vi "AlliGator Load SS1 FLI Dataset Information.vi"(8 "error in (no error)":errorcluster, 10 "Laser Period":dbl[unit], 11 "Image Folder":path) -> (0 "error out":errorcluster, 1 "Data Description":string, 2 "Metadata":string, 3 "FLI Data File Information":T1)   [LabVIEW 2021, in "AlliGator Files.lvlib"]
doc: "Loads data information from SS1 dataset."
uses:
  AlliGator Files.lvlib
  AlliGator FLI Data File Information.ctl
  Phasor/Phasor Fluorescence Lifetime Parameters v3.ctl
  AlliGator FLI Dataset Type.ctl
  AlliGator Settings List.ctl
  SwissSPAD/SwissSPAD 1 Extended Dataset Information.ctl
  SwissSPAD/SwissSPAD1 File Information.ctl
  AlliGator Load Single Gate Image from SS1 Dataset.vi
  AlliGator HDF5.lvlib
  Time/Time.lvlib
  SwissSPAD/SwissSPAD.lvlib
  AlliGator Settings.lvlib
  Phasor/Phasor.lvlib
panel:
  out "Header Size":i64
  # "see the AlliGator License on the block diagram (Ctrl+E or Window:Show Block Diagram)"
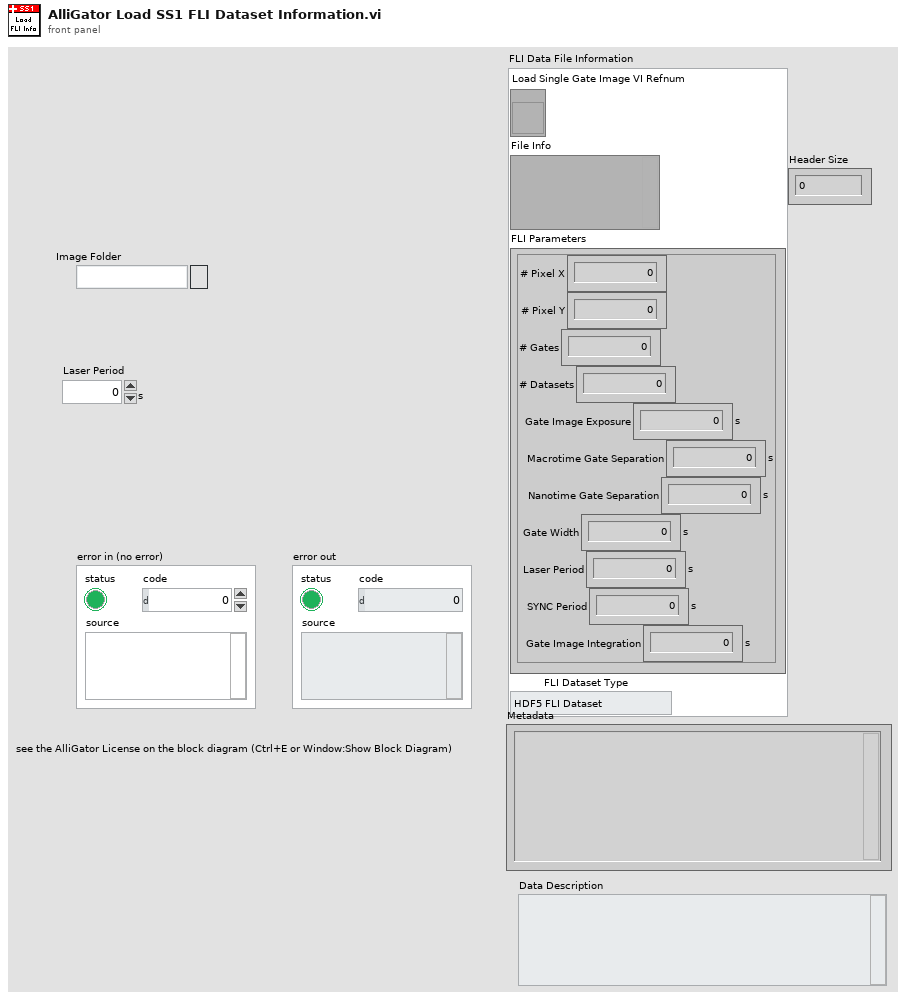
[diagram p1: front panel]
types:
  T1 = typedef "AlliGator HDF5.lvlib/AlliGator FLI Data File Information.ctl" = cluster{"Load Single Gate Image VI Refnum":refnum<vi>, "File Info":variant, "FLI Parameters":T2, "FLI Dataset Type":T3}
  T2 = typedef "Phasor.lvlib/Phasor Fluorescence Lifetime Parameters v3.ctl" = cluster{"# Pixel X":i32, "# Pixel Y":i32, "# Gates":i32, "# Datasets":i32, "Gate Image Exposure":dbl[unit], "Macrotime Gate Separation":dbl[unit], "Nanotime Gate Separation":dbl[unit], "Gate Width":dbl[unit], "Laser Period":dbl[unit], "SYNC Period":dbl[unit], "Gate Image Integration":dbl[unit]}
  T3 = typedef "AlliGator Files.lvlib/AlliGator FLI Dataset Type.ctl" = enum16{"HDF5 FLI Dataset", "Gate Image Folder", ".sdt FLI Dataset (Becker & Hickl)", ".ptu FLI Dataset (PicoQuant)", "SS1 FLI Dataset", "SS2 FLI Dataset", "I/m/phi Dataset", ".bin FLI Dataset (PicoQuant Binned)", ".bin FLI Dataset (Piccolo Binned)"}
  T4 = typedef "SwissSPAD.lvlib/SwissSPAD 1 Extended Dataset Information.ctl" = cluster{"File Path":path, "Data Offset (in bytes)":i64, "# Bytes/Pixel":i32, "# Pixel X":i32, "# Pixel Y":i32, "SwissSPAD1 File Information":T5}
  T5 = typedef "SwissSPAD.lvlib/SwissSPAD1 File Information.ctl" = cluster{"SPAD Off Pattern":u64, "Recharge Pattern":u64, "Gate Pattern":u64, "Pattern Length":u32, "# Repetitions":u32, "Initial Macro Shift":u32, "Initial Micro Shift":u32, "VOP Voltage":dbl, "Top Gate Voltage":dbl, "Bias Voltage":dbl, "# Readouts/Frame":u32, "Scan Start (step unit)":u32, "Scan Increment (step unit)":u32, "# Frames":u32, "Note":string}
  T6 = typedef "AlliGator Settings.lvlib/AlliGator Settings List.ctl" = enum16{"GUI:Visible Settings Tab", "GUI:Last Run Version", "Source Image:Use Image Histogram for Contrast", "Source Image:Low Count Pixels Rejection Options", "Source Image:High Count Pixels Rejection Options", "Source Image:Use Image Brightness", "Source Image:Blend Overlay with Image Background", "Source Image:Use Fixed ROI Diameter", "Source Image:ROI Diameter", "Source Image:ROI Center Color", "Source Image:Peak Threshold", "Source Image:Intensity Threshold", "Source Image:Image Binning Options", "Source Image:Image Smoothing Options", "Source Image:Image Histogram Active", "Source Image:Invert Binary Mask", "Source Image:Hot Pixel Removal", "Source Image:Overlay Analyzed ROI Center", "Source Image:Auto-Adjust Contrast", "Source Image:Histogram Lower Percentile", "Source Image:Histogram Upper Percentile", "Source Image:Save Source Image", "Source Image:Scale Bar Options", "Source Image:Image Resolution (Pixel Size)", "Source Image:Flatfield Correction", "Source Image:Show Dead Left Columns Correction", "Source Image:Dead Left Columns Correction", "Source Image:Image Pre-Processing Operations Order", "Data Information:Gate Width", "Data Information:Nanotime Gate Separation", "Data Information:Macrotime Gate Separation", "Data Information:Gate Step", "Data Information:# Gates", "Data Information:Gate Image Exposure", "Data Information:Gate Image Integration", "Data Information:Gates to Skip", "Data Information:Gates to Keep", "Data Information:Define Gates to", "Data Information:Channel Name", "Data Information:Available Channel Names", "Data Information:Channel Arithmetic", "Data Information:Background File Subtraction", "Data Information:Background File", "Data Information:Background Scaling Factor", "Data Information:Background Pile-up Correction", "Data Information:Background Pixel Well Capacity", "Data Information:Laser Period", "Data Information:SYNC Period", "Data Information:Pile-up Correction", "Data Information:Pixel Well Capacity", "Data Information:Dataset Scaling Factor", "Fluorescence Decay_Decay Pre-Processing:Reverse Gates", "Fluorescence Decay_Decay Pre-Processing:Verbose Decay Pre-Processing", "Fluorescence Decay_Decay Pre-Processing:Use Decay Pre-Processing", "Fluorescence Decay_Decay Pre-Processing:Background Subtraction", "Fluorescence Decay_Decay Pre-Processing:Background Definition Range", "Fluorescence Decay_Decay Pre-Processing:Baseline Subtraction Method", "Fluorescence Decay_Decay Pre-Processing:Decay Pre-Processing Operations Order", "Fluorescence Decay_Decay Pre-Processing:Smoothing Parameter", "Fluorescence Decay_Decay Pre-Processing:Shift Decay", "Fluorescence Decay_Decay Pre-Processing:Decay Shift Parameters", "Fluorescence Decay_Decay Pre-Processing:Fold Decay", "Fluorescence Decay_Decay Pre-Processing:# Folds", "Fluorescence Decay_Decay Pre-Processing:1-Normalize Decay", "Fluorescence Decay_Decay Pre-Processing:[0-1]-Normalize Decay", "Fluorescence Decay_Decay Pre-Processing:Smoothen Decay", "Fluorescence Decay_Decay Pre-Processing:Extrapolate Decay", "Fluorescence Decay_Decay Pre-Processing:Use Periodicity", "Fluorescence Decay_Decay Pre-Processing:Use Cursors", "Fluorescence Decay_Decay Pre-Processing:Tail Fraction", "Fluorescence Decay_Decay Pre-Processing:Head Fraction", "Fluorescence Decay_Decay Pre-Processing:Additional Points", "Fluorescence Decay_Decay Pre-Processing:Straighten Decay", "Fluorescence Decay_Decay Pre-Processing:Constant Background", "Fluorescence Decay_Decay Pre-Processing:Pixel-Normalize Decay", "Fluorescence Decay_Advanced Analysis:Extract IRF instead of Decay", "Fluorescence Decay_Advanced Analysis:IRF Extraction Options", "Fluorescence Decay_Advanced Analysis:IRF Optimization Options", "Fluorescence Decay_Advanced Analysis:Square Pulse Options", "Fluorescence Decay_Advanced Analysis:IRF Order", "Fluorescence Decay_Advanced Analysis:IRF Time Constants", "Fluorescence Decay_Advanced Analysis:Wavelet Analysis Options", "Fluorescence Decay_Advanced Analysis:Average Lifetime Options", "Fluorescence Decay_Fit Options:Fit Options", "Fluorescence Decay_Fit Options:Use Legacy Fitting Approach", "Fluorescence Decay_Fit Options:Use Data Information Laser Period", "Fluorescence Decay_Fit Parameters:Displayed Fit Parameters", "Fluorescence Decay_Fit Parameters:Fit Parameter Constraints", "Fluorescence Decay_Fit Parameters:Export Tabulated Results", "Fluorescence Decay_Fit Parameters:MLE Baseline Offset Type", "Fluorescence Decay_Fit Parameters:MLE Baseline Offset", "Fluorescence Decay_Fit Parameters:Guess Parameter Names", "Fluorescence Decay_Fit Parameters:Guess Parameter Values", "Fluorescence Decay_Fit Parameters:Guess Parameters Options", "Fluorescence Decay_Styles:Show Last Decay Only", "Fluorescence Decay_Styles:Decay Graph Color Array", "Fluorescence Decay:Decay Graph Active", "Fluorescence Decay Statistics:Min Peak Value", "Fluorescence Decay Statistics:Reject Low Decay Peak Pixels", "Fluorescence Decay Statistics:Reject High Decay Peak Pixels", "Fluorescence Decay Statistics:Max Peak Value", "Time Traces:Use File Timestamp", "Time Traces:Time Step", "Time Traces:Use Intensity Correction File", "Time Traces:Intensity Correction File", "Phasor Plot:Phasor Plot Smoothing Options", "Phasor Plot:Phasor Plot Size", "Phasor Plot:Phasor Plot Graphics Options", "Phasor Plot:Cumulative Phasor Plot", "Phasor Plot:Use Phasor Brightness", "Phasor Plot:Blend Overlay with Phasor Background", "Phasor Plot:Save Phasor Plot", "Phasor Plot:Show References", "Phasor Plot:Phasor Ratio Decay Range", "Phasor Plot:Exponential Fading", "Phasor Plot:Phasor Ratio Reference Colors", "Phasor Plot:Reference Radius", "Phasor Plot:Show Color Map Vertices", "Phasor Plot:Phasor Plot Active", "Phasor Plot:Phasor Ratio Color Map Type", "Phasor Plot:Phasor Ratio Color Map", "Phasor Plot:Phasor Ratio Display Range", "Phasor Plot:Selected Image ROI(s)", "Phasor Plot:All Image ROIs", "Phasor Plot:Selected Phasor Plot ROI(s)", "Phasor Plot:All Phasor Plot ROIs", "Phasor Plot:Phasor Ratio Color-Coded Quantity", "Phasor Plot:Store Phasor Harmonics", "Phasor Plot:Draw Reference Segment", "Phasor Plot:User-Defined Quantity", "Phasor Graph:Phasor Frequency", "Phasor Graph:Phasor Ratio Type", "Phasor Graph:Pixel-level Phasor Computation", "Phasor Graph:Save Phasor Graph", "Phasor Graph:Phasor Graph Active", "Phasor Graph:Phasor SDV Options", "Phasor Calibration:Use Backup Calibration if needed", "Phasor Graph:Define Shortest Lifetime as", "Phasor Calibration:Backup Calibration Type", "Phasor Calibration:Calibration Type", "Phasor Calibration:Calibration Lifetime", "Phasor Calibration:Calibration Map Algorithm", "Single-Exponential Phasor Locus (SEPL):Gate Parameters", "Single-Exponential Phasor Locus (SEPL):User-defined Gate", "Single-Exponential Phasor Locus (SEPL):User-defined IRF", "Single-Exponential Phasor Locus (SEPL):Phasor Parameters", "Single-Exponential Phasor Locus (SEPL):Decay & IRF Parameters", "Single-Exponential Phasor Locus (SEPL):Display Parameters", "Lifetime Analysis:Decay Analysis Parameters", "Lifetime Analysis:Lifetime Map Active", "Plugins:Python Settings", "Miscellaneous:Verbose Mode", "Miscellaneous:Beep after Script", "Miscellaneous:Saved Image File Format", "Miscellaneous:Exported Gate Image Settings", "Miscellaneous:Include Loading in Timing", "Miscellaneous:Verbose Settings Mode", "Miscellaneous:Histogram Options", "Miscellaneous:Beep on Error", "Miscellaneous:# Logical Processors Used", "Miscellaneous:ROI Description Max Characters", "Miscellaneous:Verbose Error Mode", "Miscellaneous:Transparent Mask Color"}
  T7 = enum16{"big-endian, network order", "native, host order", "little-endian"}
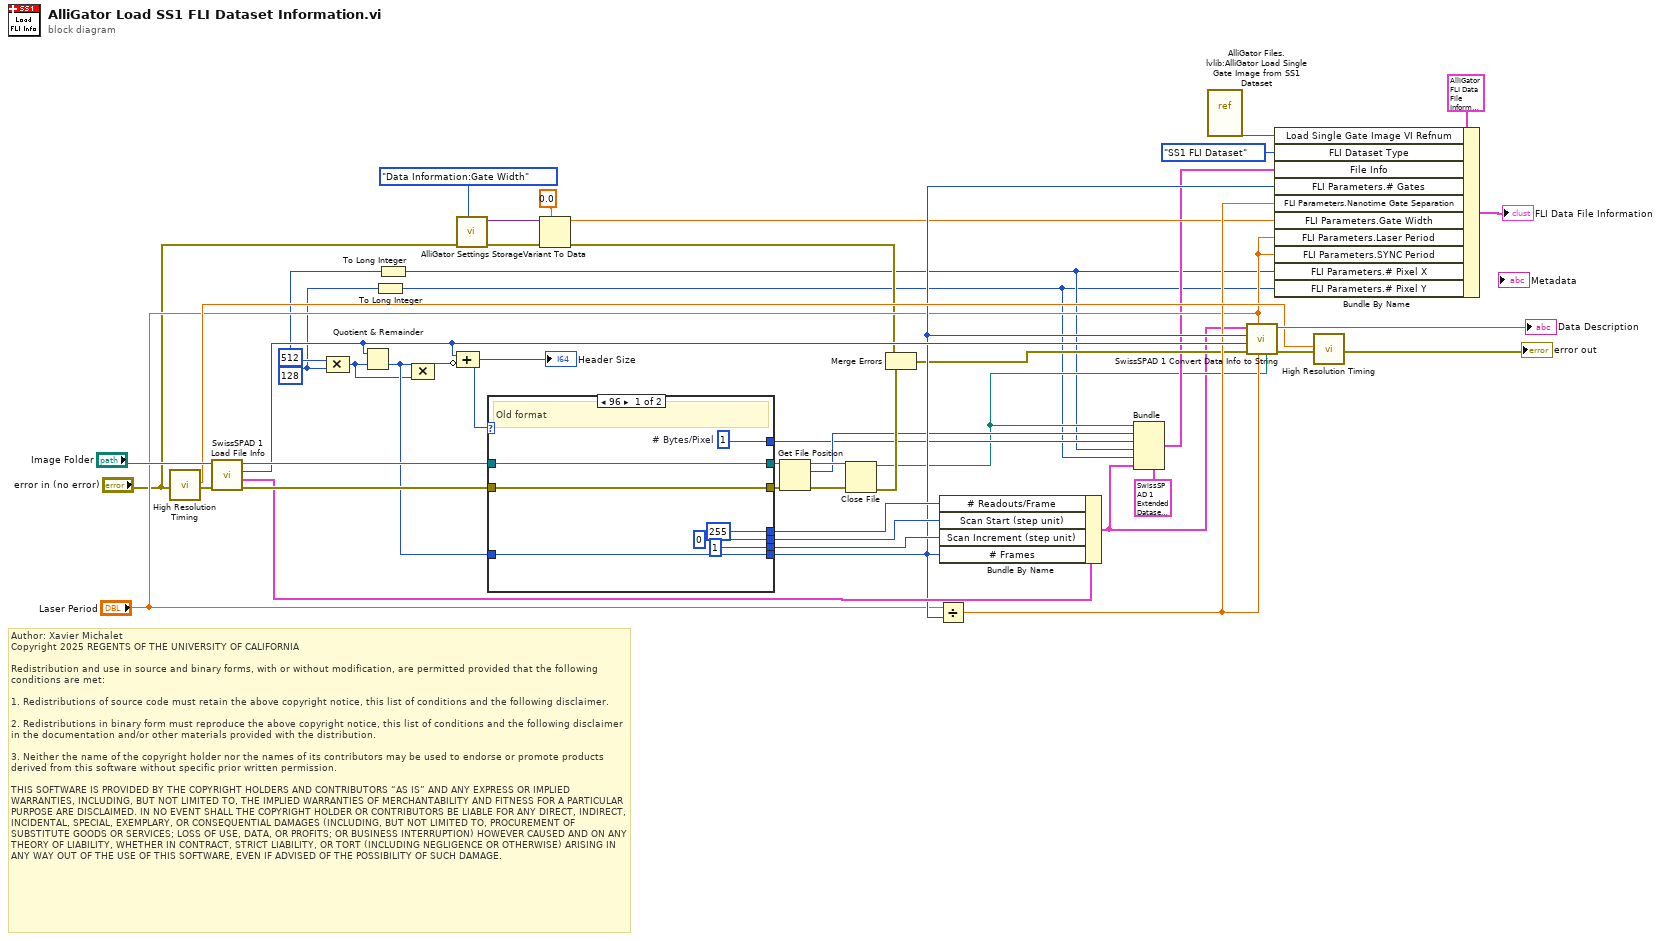
[diagram p0: block diagram]
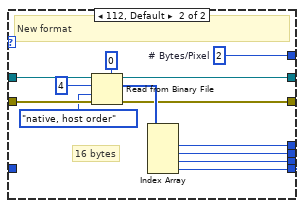
[diagram p2: hidden frame]
diagram:
  w3 = i64 128
  w4 = i64 512
  # "Author: Xavier Michalet\nCopyright 2025 REGENTS OF THE UNIVERSITY OF CALIFORNIA\n\nRedistribution and use in source and binary forms, with or without modification, are permitted provided that the following conditions are met:\n\n1. Redistributions of source code must retain the above copyright notice, this list of conditions and the following disclaimer.\n\n2. Redistributions in binary form must reproduce the above copyright notice, this list of conditions and the following disclaimer in the documentation and/or other materials provided with the distribution.\n\n3. Neither the name of the copyright holder nor the names of its contributors may be used to endorse or promote products derived from this software without specific prior written permission.\n\nTHIS SOFTWARE IS PROVIDED BY THE COPYRIGHT HOLDERS AND CONTRIBUTORS “AS IS” AND ANY EXPRESS OR IMPLIED WARRANTIES, INCLUDING, BUT NOT LIMITED TO, THE IMPLIED WARRANTIES OF MERCHANTABILITY AND FITNESS FOR A PARTICULAR PURPOSE ARE DISCLAIMED. IN NO EVENT SHALL THE COPYRIGHT HOLDER OR CONTRIBUTORS BE LIABLE FOR ANY DIRECT, INDIRECT, INCIDENTAL, SPECIAL, EXEMPLARY, OR CONSEQUENTIAL DAMAGES (INCLUDING, BUT NOT LIMITED TO, PROCUREMENT OF SUBSTITUTE GOODS OR SERVICES; LOSS OF USE, DATA, OR PROFITS; OR BUSINESS INTERRUPTION) HOWEVER CAUSED AND ON ANY THEORY OF LIABILITY, WHETHER IN CONTRACT, STRICT LIABILITY, OR TORT (INCLUDING NEGLIGENCE OR OTHERWISE) ARISING IN ANY WAY OUT OF THE USE OF THIS SOFTWARE, EVEN IF ADVISED OF THE POSSIBILITY OF SUCH DAMAGE."
  n1 = call "High Resolution Timing.vi"("Error In"="error in (no error)") -> ("elapsed (relative) seconds"=w20:dbl, "Error Out"=w29:errorcluster)  [unwired: 16 in, 1 out]
  n2 = call "SwissSPAD 1 Load File Info.vi"("error in (no error)"=w29, "File Path"="Image Folder") -> ("error out"=w40:errorcluster, "Swiss SPAD File Information"=w39:T5, "size (in bytes)"=w28:i64, "Byte Stream File out"=w41:refnum<file>)  [unwired: 6 in]
  n3 = Compound Arithmetic op=MULTIPLY(w4, w3) -> (w35:i64)
  n4 = Quotient & Remainder(x=w28, y=w35) -> (floor(x/y)=w38:i64)  [unwired: 1 out]
  n5 = To Long Integer(number=w3) -> (32bit integer=w1:i32)
  n6 = To Long Integer(number=w4) -> (32bit integer=w2:i32)
  n7 = Compound Arithmetic op=MULTIPLY(w38, w35) -> (w36:i64)
  n8 = call "AlliGator Settings Storage.vi"("AlliGator Settings List"=AlliGator_Settings_List."Data Information:Gate Width", "Error In"="error in (no error)") -> ("Error Out"=w45:errorcluster, "Variant Data out"=w44:variant)  [unwired: 8 in]
  n9 = Compound Arithmetic op=ADD(w28, invert w36) -> (w37:i64)
  "Header Size" <- w37
  n10 = case shown="96" w37 {
    tunnel: [w48 w56] -> w31
    tunnel: [w49 w57] -> w26
    tunnel: w41 -> [w49 w67]
    tunnel: w40 -> [w48 w66]
    tunnel: [u32 255 ("U32") w65] -> w32
    tunnel: [u32 0 ("U32") w64] -> w33
    tunnel: [u32 1 ("U32") w63] -> w34
    tunnel: [w51 w62] -> w19
    tunnel: w38 -> [w51 _]
    tunnel: [w50 w58] -> w9
    frame 96 {
      w50 = 1  # # Bytes/Pixel
      # "Old format"
    }
    frame 112, Default {
      w58 = 2  # # Bytes/Pixel
      # "16 bytes"
      # "New format"
      n11 = Read from Binary File(5:u32 0 ("U32"), 8:w66, 9:T7."native, host order" ("byte order (0:big-endian, network order)"), 10:4 ("count (1)"), 11:w67) -> (0:w56:errorcluster, 2:w60:u32[], 3:w57:refnum<file>)  [unwired: 1 in, 1 out]
      n12 = Index Array(array=w60) -> (element #1=w65:u32, element #2=w64:u32, element #3=w63:u32, element #4=w62:u32)  [unwired: 4 in]
    }
  }
  n13 = Variant To Data(error in=w45, type=dbl[unit] 0.0 ("Gate Duration"), Variant=w44) -> (data=w14:dbl[unit], error out=w11:errorcluster)
  n14 = Get File Position(4:w31, 7:w26) -> (0:w27:errorcluster, 2:w10:i64, 3:w25:refnum<file>)
  n15 = Close File(refnum=w25, error in=w27) -> (path=w6:path, error out=w23:errorcluster)
  n16 = Merge Errors(w11, w23) -> (w12:errorcluster)
  n17 = Divide(x="Laser Period", y=w19) -> (x/y=w16:dbl[unit])
  n18 = Bundle By Name(cluster=w39, "# Readouts/Frame"=w32, "Scan Start (step unit)"=w33, "Scan Increment (step unit)"=w34, "# Frames"=w19) -> (w5:T5)
  n19 = Bundle(cluster=T4 {"File Path"=path "", "Data Offset (in bytes)"=0, "# Bytes/Pixel"=0, "# Pixel X"=0, "# Pixel Y"=0, "SwissSPAD1 File Information"={"SPAD Off Pattern"=0, "Recharge Pattern"=0, "Gate Pattern"=0, "Pattern Length"=0, "# Repetitions"=0, "Initial Macro Shift"=0, "Initial Micro Shift"=0, "VOP Voltage"=0.0, "Top Gate Voltage"=0.0, "Bias Voltage"=0.0, "# Readouts/Frame"=0, "Scan Start (step unit)"=0, "Scan Increment (step unit)"=0, "# Frames"=0, "Note"=""}} ("output cluster"), "File Path"=w6, "Data Offset (in bytes)"=w10, "# Bytes/Pixel"=w9, "# Pixel X"=w2, "# Pixel Y"=w1, "SwissSPAD1 File Information"=w5) -> (w8:T4)
  n20 = vi-ref "AlliGator Files.lvlib:AlliGator Load Single Gate Image from SS1 Dataset.vi"() -> (w17:refnum<vi>)
  n21 = call "SwissSPAD 1 Convert Data Info to String.vi"("File Path"=w6, "Step Duration"=w16, "Laser Period"="Laser Period", "error in (no error)"=w12, "size"=w28, "# Frames"=w19, "Swiss SPAD 1 File Information"=w5) -> ("Error Out"=w22:errorcluster, "Data Description"=→"Data Description":string)  [unwired: 3 in]
  n22 = Bundle By Name(cluster=T1 {"Load Single Gate Image VI Refnum"=refnum, "File Info"=variant, "FLI Parameters"={"# Pixel X"=0, "# Pixel Y"=0, "# Gates"=0, "# Datasets"=0, "Gate Image Exposure"=0.0, "Macrotime Gate Separation"=0.0, "Nanotime Gate Separation"=0.0, "Gate Width"=0.0, "Laser Period"=0.0, "SYNC Period"=0.0, "Gate Image Integration"=0.0}, "FLI Dataset Type"=enum."HDF5 FLI Dataset"} ("FLI Data File Information"), "Load Single Gate Image VI Refnum"=w17, "FLI Dataset Type"=AlliGator_FLI_Dataset_Type."SS1 FLI Dataset", "File Info"=w8, "FLI Parameters.# Gates"=w19, "FLI Parameters.Nanotime Gate Separation"=w16, "FLI Parameters.Gate Width"=w14, "FLI Parameters.Laser Period"="Laser Period", "FLI Parameters.SYNC Period"="Laser Period", "FLI Parameters.# Pixel X"=w2, "FLI Parameters.# Pixel Y"=w1) -> (→"FLI Data File Information":T1)
  n23 = call "High Resolution Timing.vi"("relative seconds (NaN)"=w20, "Error In"=w22) -> ("Error Out"=→"error out":errorcluster)  [unwired: 15 in, 2 out]
